vi "json Insert Float - array path.vi"(8 "error in (no error)":errorcluster, 9 "anything":sgl, 10 "path":string[](array[string]), 11 "JSON Document in":refnum<class "JSON Document.lvclass">) -> (0 "error out":errorcluster, 3 "JSON Document out":refnum<class "JSON Document.lvclass">)   [LabVIEW 2015, in "JSON Document.lvclass"]
uses:
  JSON Document.lvclass
  json Insert Float - string path.vi
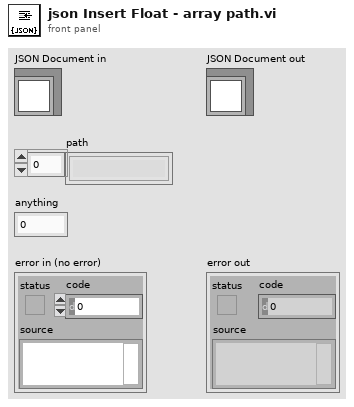
[diagram p1: front panel]
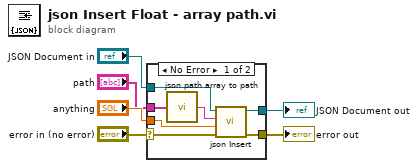
[diagram p0: block diagram]
diagram:
  n1 = case shown="No Error" "error in (no error)" {
    selector: "error in (no error)" -> [w7 w15]
    tunnel: [w11 w15] -> w5
    tunnel: [w10 w14] -> w3
    tunnel: "JSON Document in" -> [w9 w14]
    tunnel: "anything" -> [w8 _]
    tunnel: "path" -> [w12 _]
    frame No Error {
      n2 = call "json path array to path.vi"("path"=w12) -> ("String"=w13:string)
      n3 = call-poly "json Insert.vi"("error in (no error)"=w7, "anything"=w8, "path"=w13, "JSON Document in"=w9) -> ("error out"=w11:errorcluster, "JSON Document out"=w10:refnum<class "JSON Document.lvclass">)  [unwired: 6 in]
    }
    frame Error {
    }
  }
  "error out" <- w5
  "JSON Document out" <- w3
